vi "Subtraction.vi"() -> ()   [LabVIEW 2018]
doc: "Use this template to build a VI to use as a subVI."
uses:
  <vilib>/vision/NI_Vision_Development_Module.lvlib
panel:
  out "SrcB":T1(plugin-control)
  out "SrcA":T1(plugin-control)
  out "Dst":T1(plugin-control)
  # ":: MVi Framework V1.0 ::\nAuthor:Gaoke Yang\nEmail: gaoke.yang@yahoo.com\nWeb: www.mvicontrol.com\nCopyright (C) 2015, MVI Technologies All Rights Reserved"
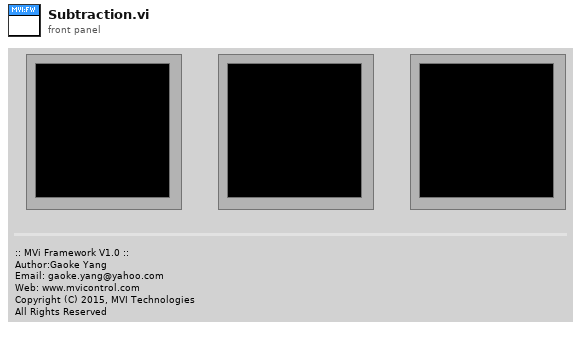
[diagram p1: front panel]
types:
  T1 = typedef "IMAQ Image.ctl" = refnum<image>
  T2 = typedef "Image Type" = u32
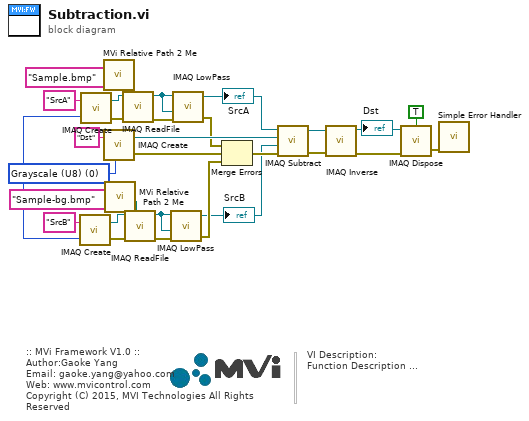
[diagram p0: block diagram]
diagram:
  w15 = T2 0 items=["Grayscale (U8)", "Grayscale (I16)", "Grayscale (SGL)", "Complex (CSG)", "RGB (U32)", "HSL (U32)", "RGB (U64)", "Grayscale (U16)"] ("Image Type")
  # "VI Description:\nFunction Description ..."
  # ":: MVi Framework V1.0 ::\nAuthor:Gaoke Yang\nEmail: gaoke.yang@yahoo.com\nWeb: www.mvicontrol.com\nCopyright (C) 2015, MVI Technologies All Rights Reserved"
  n1 = call "IMAQ Create"("Image Name"="SrcB" ("name or relative path"), "Image Type"=w15) -> ("New Image"=w20:T1, "error out"=w17:errorcluster)  [unwired: 2 in, 1 out]
  n2 = call "IMAQ Create"("Image Name"="SrcA" ("name or relative path"), "Image Type"=w15) -> ("New Image"=w22:T1, "error out"=w25:errorcluster)  [unwired: 2 in, 1 out]
  n3 = call "MVi Relative Path 2 Me.vi"("Relative Path"="Sample.bmp" ("name or relative path")) -> ("Appended Dir"=w23:path)  [unwired: 5 in, 1 out]
  n4 = call "IMAQ Create"("Image Name"="Dst" ("name or relative path"), "Image Type"=w15) -> ("New Image"=w13:T1, "error out"=w21:errorcluster)  [unwired: 2 in, 1 out]
  n5 = call "MVi Relative Path 2 Me.vi"("Relative Path"="Sample-bg.bmp" ("name or relative path")) -> ("Appended Dir"=w19:path)  [unwired: 5 in, 1 out]
  n6 = call "IMAQ ReadFile"("File Path"=w23, "error in (no error)"=w25, "Image"=w22) -> ("error out"=w8:errorcluster, "Image Out"=w7:T1)  [unwired: 4 in, 3 out]
  n7 = call "IMAQ ReadFile"("File Path"=w19, "error in (no error)"=w17, "Image"=w20) -> ("error out"=w5:errorcluster, "Image Out"=w4:T1)  [unwired: 4 in, 3 out]
  n8 = call "IMAQ LowPass"("Image Src"=w4, "Image Dst"=w4, "error in (no error)"=w5) -> ("Image Dst Out"=w1:T1, "error out"=w2:errorcluster)  [unwired: 4 in]
  "SrcB" <- w1
  n9 = call "IMAQ LowPass"("Image Src"=w7, "Image Dst"=w7, "error in (no error)"=w8) -> ("Image Dst Out"=w6:T1, "error out"=w3:errorcluster)  [unwired: 4 in]
  "SrcA" <- w6
  n10 = Merge Errors(w3, w21, w2) -> (w14:errorcluster)
  n11 = call "IMAQ Subtract"("Image Src A"=w6, "Image Dst"=w13, "Image Src B"=w1, "error in (no error)"=w14) -> ("Image Dst Out"=w10:T1, "error out"=w12:errorcluster)  [unwired: 3 in]
  n12 = call "IMAQ Inverse"("error in (no error)"=w12, "Image Src"=w10) -> ("error out"=w11:errorcluster, "Image Dst Out"=w9:T1)  [unwired: 8 in]
  "Dst" <- w9
  n13 = call "IMAQ Dispose"("All Images? (No)"=TRUE, "Image"=w9, "error in (no error)"=w11) -> ("error out"=w28:errorcluster)  [unwired: 3 out]
  n14 = call <vilib>:"Simple Error Handler.vi"("error in (no error)"=w28) -> ()  [unwired: 1 in, 8 out]
